vi "VisFrmWrkRequestingVisStop.vi"(8 "error in (no error)":errorcluster, 10 "VisualizationPluginNameToStop":string) -> (0 "error out":errorcluster)   [LabVIEW 2018, in "Visualization.lvlib" / "VisualizeBase.lvclass"]
uses:
  VisualizeBase.lvclass
  Scope/ScopeShared/clEventType.ctl
  Scope/ScopeShared/ScopeShared.lvlib
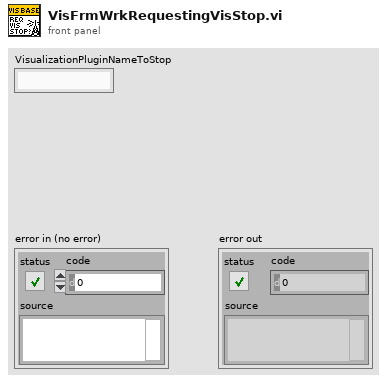
[diagram p1: front panel]
types:
  T1 = typedef "ScopeShared.lvlib/clEventType.ctl" = cluster{"ModuleID":i32, "Data":variant}
  T2 = typedef "Visualization.lvlib/VisualizeBase.lvclass/VisFrmWrkBroadcastEvents.ctl" = cluster{"StatusUpdate":refnum<user-event>, "DidStop":refnum<user-event>, "NewModuleLoaded":refnum<user-event>, "StopVisualization":refnum<user-event>}
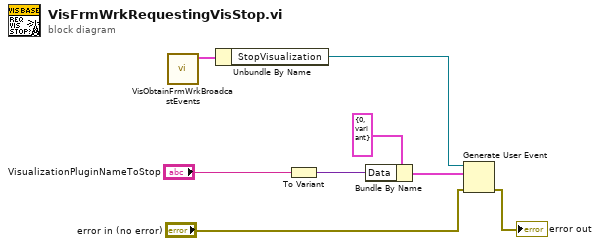
[diagram p0: block diagram]
diagram:
  n1 = call "VisObtainFrmWrkBroadcastEvents.vi"() -> ("VisFrmWrkBroadcastEvents"=w4:T2)  [unwired: 10 in, 1 out]
  n2 = Unbundle By Name(w4) -> ("StopVisualization"=w8:refnum<user-event>)
  n3 = To Variant(anything="VisualizationPluginNameToStop") -> (Variant=w7:variant)
  n4 = Bundle By Name(cluster=T1 {"ModuleID"=0, "Data"=variant} ("event data"), "Data"=w7) -> (w1:T1)
  n5 = Generate User Event(user event=w8, event data cluster=w1, error in="error in (no error)") -> (error out=→"error out":errorcluster)  [unwired: 1 in, 1 out]
